vi "XIPIN_Mailbox_2_1.vi"   [LabVIEW 2017]
doc: "Mailbox Interprocessor Communication\n------------------------------------\n<b>Need License</b> : No\n<b>Interface</b> : AXI4 AXI4-Stream"
uses:
  <vilib>/rvi/XilinxIP/XIPIN_XNode/niFpgaXIPIN.xnode
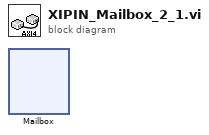
[diagram p0: block diagram]
diagram:
  n1 = xnode ("Mailbox")() -> ()
